vi "Configure Acquisition Sample.vi"(8 "error in (no error)":errorcluster, 9 "Averages (4)":dbl=4.0, 10 "Acquisition (0: Sampling)":u16(ring) items=["Sampling", "Peak_Detect", "Average"], 11 "VISA resource name":refnum<visa-resource-name>) -> (0 "error out":errorcluster, 3 "VISA resource name out":refnum<visa-resource-name>)   [LabVIEW 2021, in "Siglent SDS 1000 2000 Series.lvlib"]
doc: "Controls the sample mode of the instrument. Choices are Sampling, Peak Detect and Average. Not all modes are available, depending upon the scope model, timebase setting, etc."
uses:
  <instrlib>/Siglent SDS 1000 2000 Series/Siglent SDS 1000 2000 Series.lvlib
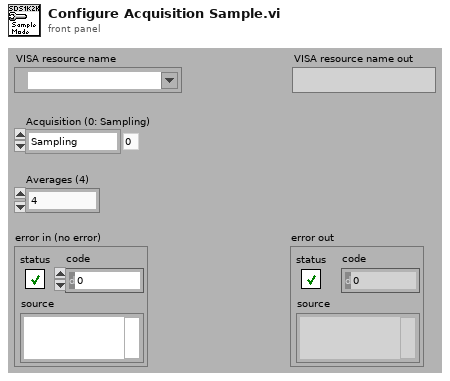
[diagram p1: front panel]
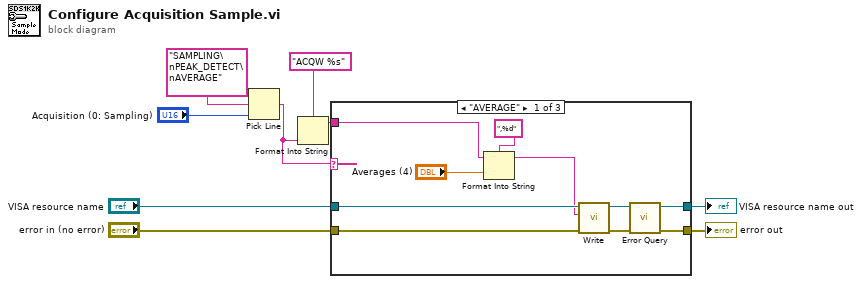
[diagram p0: block diagram]
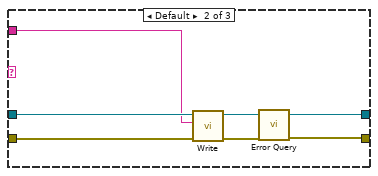
[diagram p2: hidden frame]
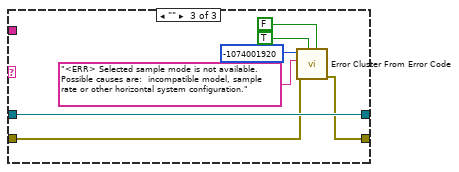
[diagram p3: hidden frame]
diagram:
  n1 = Pick Line(multi-line string="SAMPLING\nPEAK_DETECT\nAVERAGE", line index="Acquisition (0: Sampling)") -> (output string=w1:string)  [unwired: 1 in]
  n2 = Format Into String(format string="ACQW %s", w1) -> (resulting string=w9:string)  [unwired: 2 in, 1 out]
  n3 = case shown="\"AVERAGE\"" w1 {
    tunnel: "VISA resource name" -> [w19 w26 w33]
    tunnel: "error in (no error)" -> [w18 w25 w27]
    tunnel: w9 -> [w13 w24 _]
    tunnel: [w15 w21 w33] -> w6
    tunnel: [w16 w22 w28] -> w7
    frame "AVERAGE" {
      n4 = Format Into String(format string=",%d", initial string=w13, "Averages (4)") -> (resulting string=w10:string)  [unwired: 1 in, 1 out]
      n5 = call <instrlib>:"Write.vi"("error in (no error)"=w18, "Write Buffer"=w10, "VISA resource name"=w19) -> ("error out"=w17:errorcluster, "VISA resource name out"=w14:refnum<visa-resource-name>)  [unwired: 6 in, 1 out]
      n6 = call <instrlib>:"Error Query.vi"("error in (no error)"=w17, "VISA resource name"=w14) -> ("error out"=w16:errorcluster, "VISA resource name out"=w15:refnum<visa-resource-name>)  [unwired: 6 in, 2 out]
    }
    frame Default {
      n7 = call <instrlib>:"Write.vi"("error in (no error)"=w25, "Write Buffer"=w24, "VISA resource name"=w26) -> ("error out"=w23:errorcluster, "VISA resource name out"=w20:refnum<visa-resource-name>)  [unwired: 6 in, 1 out]
      n8 = call <instrlib>:"Error Query.vi"("error in (no error)"=w23, "VISA resource name"=w20) -> ("error out"=w22:errorcluster, "VISA resource name out"=w21:refnum<visa-resource-name>)  [unwired: 6 in, 2 out]
    }
    frame "" {
      n9 = call <vilib>:"Error Cluster From Error Code.vi"("is warning? (False)"=FALSE, "show call chain? (False)"=TRUE, "error in (no error)"=w27, "error message (\"\")"="<ERR> Selected sample mode is not available. Possible causes are:  incompatible model, sample rate or other horizontal system configuration." ("source"), "error code (0)"=-1074001920 ("code")) -> ("error out"=w28:errorcluster)  [unwired: 4 in]
    }
  }
  "VISA resource name out" <- w6
  "error out" <- w7
